vi "Generate DO ReadStatus Event.vi"(8 "error in (no error)":errorcluster, 9 "DO IOName":string, 10 "CmdMsg":string="DORead_Status", 11 "DAQ":refnum<class "DAQ.lvclass">) -> (0 "error out":errorcluster, 3 "DAQ":refnum<class "DAQ.lvclass">)   [LabVIEW 2022 SP3, in "DAQ.lvclass"]
doc: "Developed by Kevin Thompson\nkevin@thompsonengineering.net\n\nCopyright 2018-2020\nThompson Engineering, LLC"
uses:
  DAQ.lvclass
  DAQ.lvclass/DAQ.ctl
  Common/Controls/TD Async CmdMsg EventData--cluster.ctl
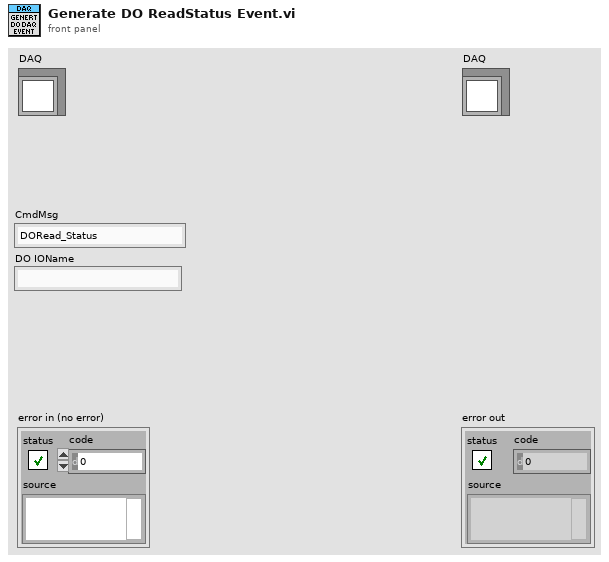
[diagram p1: front panel]
types:
  T1 = typedef "TD Async CmdMsg EventData--cluster.ctl" = cluster{"Time Stamp":timestamp, "CmdMsg":string, "vData":variant}
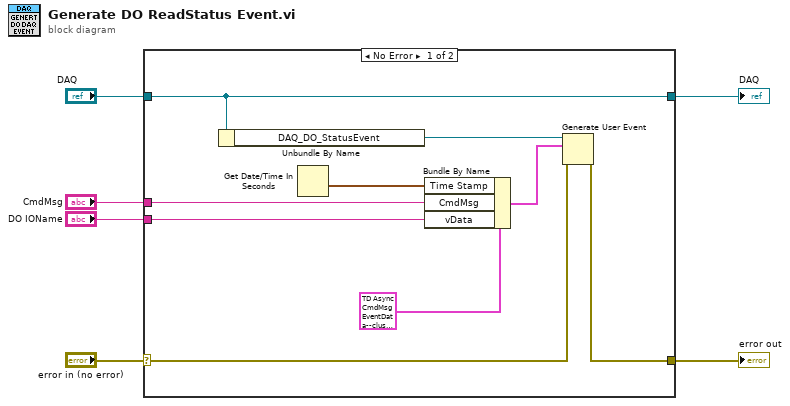
[diagram p0: block diagram]
diagram:
  n1 = case shown="No Error" "error in (no error)" {
    selector: "error in (no error)" -> [w13 w17]
    tunnel: [w12 w17] -> w5
    tunnel: [w15 w16] -> w3
    tunnel: "DAQ" -> [w15 w16]
    tunnel: "DO IOName" -> [w8 _]
    tunnel: "CmdMsg" -> [w7 _]
    frame No Error {
      n2 = Unbundle By Name(w15) -> ("DAQ_DO_StatusEvent"=w14:refnum<user-event>)
      n3 = Get Date/Time In Seconds() -> (seconds since 1Jan1904=w9:timestamp)
      n4 = Bundle By Name(cluster=T1 {"Time Stamp"=timestamp(0 s since 1904-01-01), "CmdMsg"="", "vData"=variant} ("event data"), "Time Stamp"=w9, "CmdMsg"=w7, "vData"=w8) -> (w10:T1)
      n5 = Generate User Event(user event=w14, event data cluster=w10, error in=w13) -> (error out=w12:errorcluster)  [unwired: 1 in, 1 out]
    }
    frame Error {
    }
  }
  "error out" <- w5
  "DAQ" <- w3
